vi "CommonVIs_AlignToConnectorPane.vi"(8 "error in (no error)":errorcluster, 11 "VI Ref":refnum<vi>) -> (0 "error out":errorcluster)   [LabVIEW 2020]
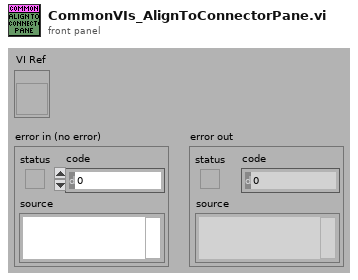
[diagram p1: front panel]
types:
  T1 = enum32{"Top Edges", "Vertical Centers", "Bottom Edges", "Left Edges", "Horizontal Centers", "Right Edges"}
  T2 = typedef "LVRectTypeDef.ctl" = cluster{"Left":i16, "Top":i16, "Right":i16, "Bottom":i16}
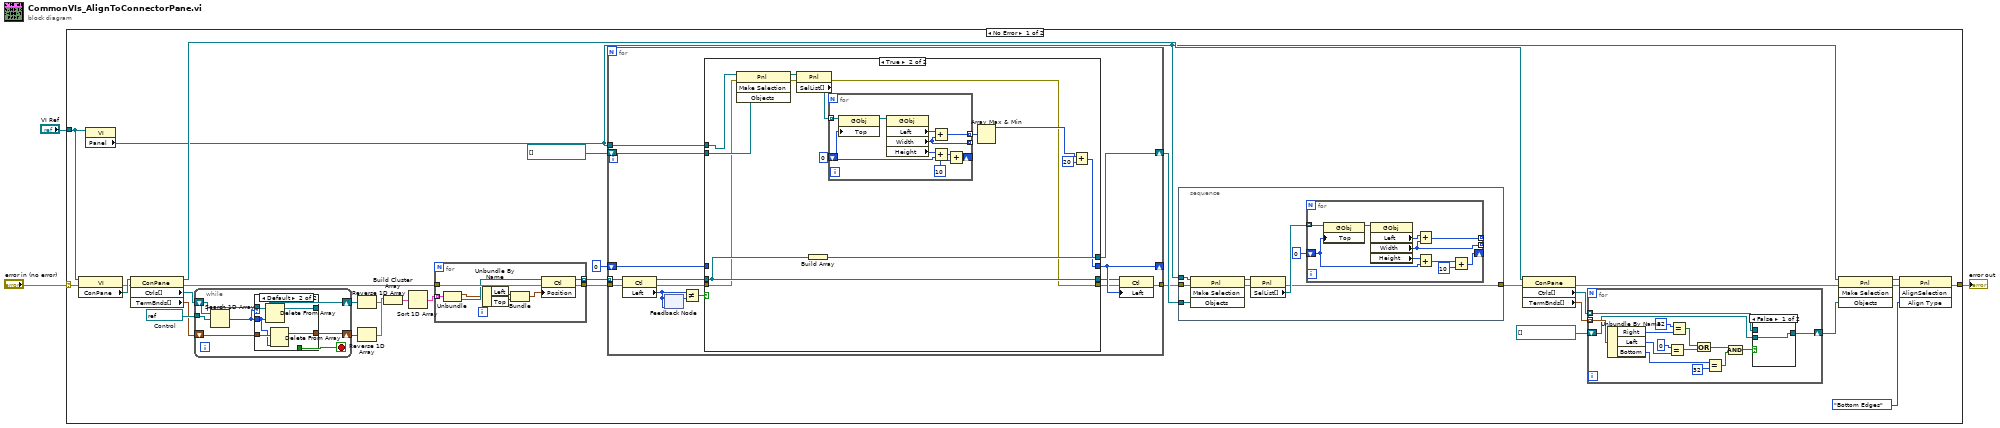
[diagram p0: block diagram]
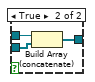
[diagram p2: hidden frame]
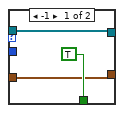
[diagram p3: hidden frame]
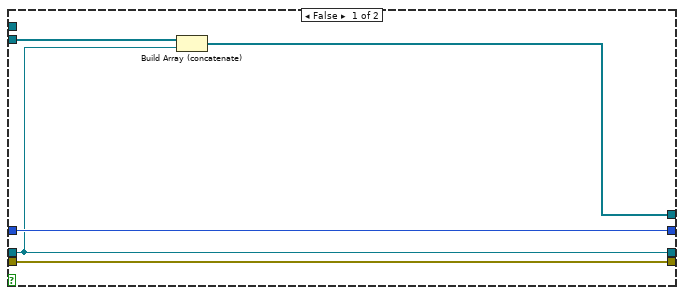
[diagram p4: hidden frame]
diagram:
  n1 = case shown="No Error" "error in (no error)" {
    selector: "error in (no error)" -> [w4 w141]
    tunnel: [w6 w141] -> w2
    tunnel: "VI Ref" -> [w5 _]
    frame No Error {
      w24 = refnum<vi> refnum  # Control
      n2 = property class="VI"(reference=w5, error in=w4) -> (error out=w30:errorcluster, "ConPane"=w32:refnum<vi>)  [unwired: 1 out]
      n3 = property class="VI"(reference=w5) -> ("Panel"=w8:refnum<vi>)  [unwired: 1 in, 2 out]
      n4 = property class="ConPane"(reference=w32, error in=w30) -> (reference out=w9:refnum<vi>, error out=w29:errorcluster, "Ctrls[]"=w23:refnum<vi>[], "TermBnds[]"=w22:T2[])
      n5 = while {
        tunnel: w24 -> [w73]
        shift-right: [w78] -> w21
        shift-left: w23 -> [w79]
        shift-right: [w74] -> w20
        shift-left: w22 -> [w75]
        stop <- w76 stop-if-true
        n6 = Search 1D Array(1D array=w79, element=w73) -> (index of element=w77:i32)  [unwired: 1 in]
        n7 = case shown="Default" w77 {
          tunnel: w77 -> [_ w83]
          tunnel: w79 -> [w82 w87]
          tunnel: [w82 w86] -> w78
          tunnel: [TRUE _] -> w76
          tunnel: w75 -> [w80 w85]
          tunnel: [w80 w84] -> w74
          frame -1 {
          }
          frame Default {
            n8 = Delete From Array(array=w87, index=w83) -> (array with subset deleted=w86:refnum<vi>[])  [unwired: 1 in, 1 out]
            n9 = Delete From Array(array=w85, index=w83) -> (array with subset deleted=w84:T2[])  [unwired: 1 in, 1 out]
          }
        }
      }
      n10 = Reverse 1D Array(array=w21) -> (reversed array=w27:refnum<vi>[])
      n11 = Reverse 1D Array(array=w20) -> (reversed array=w28:T2[])
      n12 = Build Cluster Array(w28, w27) -> (w26:cluster{"Rectangle":T2, refnum<vi>}[])
      n13 = Sort 1D Array(array=w26) -> (sorted array=w25:cluster{"Rectangle":T2, refnum<vi>}[])
      n14 = for {
        tunnel: [w93] -> w34 mode=indexing
        tunnel: [w92] -> w31
        tunnel: w29 -> [w91]
        tunnel: w25 -> [w90] mode=indexing
        n15 = Unbundle(w90) -> ("Rectangle"=w88:T2, w89:refnum<vi>)
        n16 = Unbundle By Name(w88) -> ("Left"=w96:i16, "Top"=w95:i16)
        n17 = Bundle("Left"=w96, "Top"=w95) -> (w94:cluster{"Left":i16, "Top":i16})  [unwired: 1 in]
        n18 = property class="Ctl"(reference=w89, error in=w91, "Position"=w94) -> (reference out=w93:refnum<vi>, error out=w92:errorcluster)
      }
      n19 = for {
        shift-right: [w110] -> w19
        shift-left: refnum<vi>[] [] -> [w109]
        shift-right: [w103] -> _
        shift-left: u32 0 ("Numeric") -> [w104]
        tunnel: w8 -> [w108]
        tunnel: w34 -> [w107] mode=indexing
        tunnel: [w101] -> w18
        tunnel: w31 -> [w99]
        n20 = property class="Ctl"(reference=w107, error in=w99) -> (reference out=w98:refnum<vi>, error out=w100:errorcluster, "Left"=w105:i32)
        n21 = feedback-in #1(w105) -> ()
        n22 = feedback #1(w105) -> (w111:i32)
        n23 = Not Equal?(x=w105, y=w111) -> (x != y?=w106:bool)
        n24 = case shown="True" w106 {
          tunnel: [w116 w130] -> w110
          tunnel: w109 -> [w115 w122]
          tunnel: [w114 w128] -> w103
          tunnel: w108 -> [_ w121]
          tunnel: w104 -> [w114 _]
          tunnel: [w113 w117] -> w102
          tunnel: w100 -> [w113 w118]
          tunnel: w98 -> [w112 w129]
          tunnel: [w112 w129] -> w97
          frame False {
            n25 = Build Array (concatenate)(w115, w112) -> (w116:refnum<vi>[])
          }
          frame True {
            n26 = invoke class="Pnl" method="Make Selection"(reference=w121, error in=w118, "Objects"=w122) -> (reference out=w126:refnum<vi>, error out=w125:errorcluster)  [unwired: 1 in, 2 out]
            n27 = property class="Pnl"(reference=w126, error in=w125) -> (error out=w117:errorcluster, "SelList[]"=w120:refnum<vi>[])  [unwired: 1 out]
            n28 = Build Array(w129) -> (w130:refnum<vi>[])
            n29 = for {
              tunnel: w120 -> [w133] mode=indexing
              tunnel: [w140] -> w123 mode=indexing
              tunnel: [w139] -> _ mode=indexing
              shift-right: [w134] -> _
              shift-left: u32 0 -> [w131]
              n30 = property class="GObj"(reference=w133, "Top"=w131) -> (reference out=w132:refnum<vi>)  [unwired: 1 in, 1 out]
              n31 = property class="GObj"(reference=w132) -> ("Left"=w138:i32, "Width"=w139:u32, "Height"=w137:u32)  [unwired: 1 in, 2 out]
              n32 = Add(x=w138, y=w139) -> (x+y=w140:u32)
              n33 = Add(x=w137, y=w131) -> (x+y=w136:u32)
              n34 = Add(x=w136, y=u32 10) -> (x+y=w134:u32)
            }
            n35 = Array Max & Min(array=w123) -> (max value=w119:u32)  [unwired: 3 out]
            n36 = Add(x=w119, y=u32 20) -> (x+y=w128:u32)
          }
        }
        n37 = property class="Ctl"(reference=w97, error in=w102, "Left"=w103) -> (error out=w101:errorcluster)  [unwired: 1 out]
      }
      n38 = stacked-sequence {
        tunnel: w19 -> [w58]
        tunnel: w8 -> [w57]
        tunnel: w18 -> [w56]
        tunnel: [w55] -> w7
        frame #0 {
          n39 = invoke class="Pnl" method="Make Selection"(reference=w57, error in=w56, "Objects"=w58) -> (reference out=w62:refnum<vi>, error out=w61:errorcluster)  [unwired: 1 in, 2 out]
          n40 = property class="Pnl"(reference=w62, error in=w61) -> (error out=w55:errorcluster, "SelList[]"=w59:refnum<vi>[])  [unwired: 1 out]
          n41 = for {
            tunnel: w59 -> [w65] mode=indexing
            tunnel: [w72] -> _ mode=indexing
            tunnel: [w71] -> _ mode=indexing
            shift-right: [w66] -> _
            shift-left: u32 0 -> [w63]
            n42 = property class="GObj"(reference=w65, "Top"=w63) -> (reference out=w64:refnum<vi>)  [unwired: 1 in, 1 out]
            n43 = property class="GObj"(reference=w64) -> ("Left"=w70:i32, "Width"=w71:u32, "Height"=w69:u32)  [unwired: 1 in, 2 out]
            n44 = Add(x=w70, y=w71) -> (x+y=w72:u32)
            n45 = Add(x=w69, y=w63) -> (x+y=w68:u32)
            n46 = Add(x=w68, y=u32 10) -> (x+y=w66:u32)
          }
        }
      }
      n47 = property class="ConPane"(reference=w9, error in=w7) -> (error out=w17:errorcluster, "Ctrls[]"=w10:refnum<vi>[], "TermBnds[]"=w11:T2[])  [unwired: 1 out]
      n48 = for {
        tunnel: w10 -> [w39] mode=indexing
        tunnel: w11 -> [w50] mode=indexing
        shift-right: [w38] -> w13
        shift-left: refnum<vi>[] [] -> [w37]
        n49 = Unbundle By Name(w50) -> ("Right"=w45:i16, "Left"=w47:i16, "Bottom"=w49:i16)
        n50 = Equal?(x=i16 0, y=w47) -> (x = y?=w42:bool)
        n51 = Equal?(x=i16 32 ("right"), y=w45) -> (x = y?=w43:bool)
        n52 = Or(x=w43, y=w42) -> (x .or. y?=w41:bool)
        n53 = Equal?(x=w49, y=i16 32) -> (x = y?=w40:bool)
        n54 = And(x=w41, y=w40) -> (x .and. y?=w36:bool)
        n55 = case shown="False" w36 {
          tunnel: w39 -> [_ w54]
          tunnel: [w51 w53] -> w38
          tunnel: w37 -> [w51 w52]
          frame False {
          }
          frame True {
            n56 = Build Array (concatenate)(w54, w52) -> (w53:refnum<vi>[])
          }
        }
      }
      n57 = invoke class="Pnl" method="Make Selection"(reference=w8, error in=w17, "Objects"=w13) -> (reference out=w14:refnum<vi>, error out=w16:errorcluster)  [unwired: 1 in, 2 out]
      n58 = invoke class="Pnl" method="AlignSelection"(reference=w14, error in=w16, "Align Type"=T1."Bottom Edges") -> (error out=w6:errorcluster)  [unwired: 1 in, 3 out]
    }
    frame Error {
    }
  }
  "error out" <- w2
